vi "T7 Simulator Checksum KAG.vi"() -> ()   [LabVIEW 2015]
panel:
  out "CheckLength Error":bool
  in  "Numeric":u32
  out "Array Output":u8[](array[numeric])=[139, 242, 0, 160, 247, 0]
  in  "stop":bool
  in  "Radix Control":u16(ring) items=["Decimal", "Scientific", "Engineering", "Binary", "Octal", "Hexadecimal", "Relative Time", "Date & Time", "SI"]
  out "Array Input":u8[](array[numeric])
  out "Input Checksum16 LSB":u8
  out "Calculated Checksum16 LSB":u8
  out "Input Checksum16 MSB":u8
  out "Calculated Checksum16 MSB":u8
  out "Input Checksum8":u8
  out "Calculated Checksum8":u8
  out "Checksum Error":bool
  # "Checksum8"
  # "Checksum16 LSB"
  # "Checksum16 MSB"
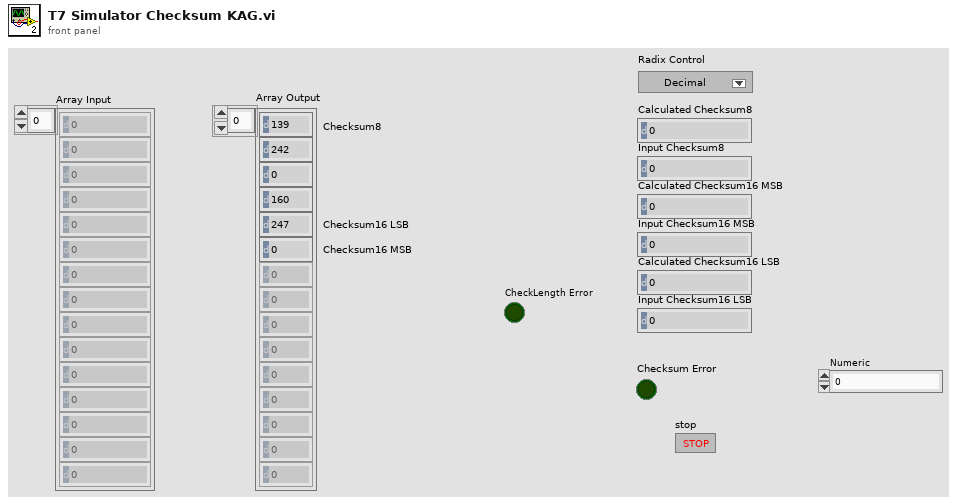
[diagram p1: front panel]
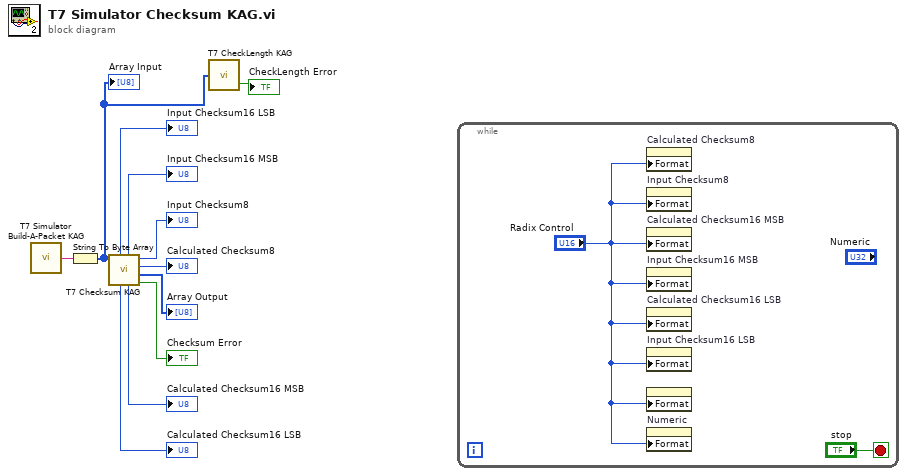
[diagram p0: block diagram]
diagram:
  n1 = call "T7 Simulator Build-A-Packet KAG.vi"() -> ("Simulated Data Packet"=w11:string)  [unwired: 10 in]
  n2 = String To Byte Array(string=w11) -> (unsigned byte array=w2:u8[])
  "Array Input" <- w2
  n3 = call "T7 Checksum KAG.vi"("Array"=w2) -> ("Checksum Error"=→"Checksum Error":bool, "Array Output"=→"Array Output":u8[], "Calculated Checksum8"=→"Calculated Checksum8":u8, "Input Checksum8"=→"Input Checksum8":u8, "Calculated Checksum16 MSB"=→"Calculated Checksum16 MSB":u8, "Input Checksum16 MSB"=→"Input Checksum16 MSB":u8, "Calculated Checksum16 LSB"=→"Calculated Checksum16 LSB":u8, "Input Checksum16 LSB"=→"Input Checksum16 LSB":u8)  [unwired: 3 in]
  n4 = call "T7 CheckLength KAG.vi"("Array"=w2) -> ("CheckLength Error"=→"CheckLength Error":bool)  [unwired: 1 out]
  n5 = while {
    stop <- "stop" stop-if-true
    n6 = property on="Calculated Checksum8" class="DigNum (strict)"("Format"="Radix Control") -> ()  [unwired: 2 in, 2 out]
    n7 = property on="Input Checksum8" class="DigNum (strict)"("Format"="Radix Control") -> ()  [unwired: 2 in, 2 out]
    n8 = property on="Calculated Checksum16 MSB" class="DigNum (strict)"("Format"="Radix Control") -> ()  [unwired: 2 in, 2 out]
    n9 = property on="Input Checksum16 MSB" class="DigNum (strict)"("Format"="Radix Control") -> ()  [unwired: 2 in, 2 out]
    n10 = property on="Calculated Checksum16 LSB" class="DigNum (strict)"("Format"="Radix Control") -> ()  [unwired: 2 in, 2 out]
    n11 = property on="Input Checksum16 LSB" class="DigNum (strict)"("Format"="Radix Control") -> ()  [unwired: 2 in, 2 out]
    n12 = property class="DigNum (strict)"("Format"="Radix Control") -> ()  [unwired: 2 in, 2 out]
    n13 = property on="Numeric" class="DigNum (strict)"("Format"="Radix Control") -> ()  [unwired: 2 in, 2 out]
  }
